vi "Generate Error.vi"(0 "Application in":refnum<class "Application.lvclass">, 5 "error in (no error)":errorcluster) -> (14 "Application out":refnum<class "Application.lvclass">)   [LabVIEW 2019, in "Application.lvclass"]
uses:
  Application.lvclass
  ErrorEvent.ctl
  Application.lvclass/Application.ctl
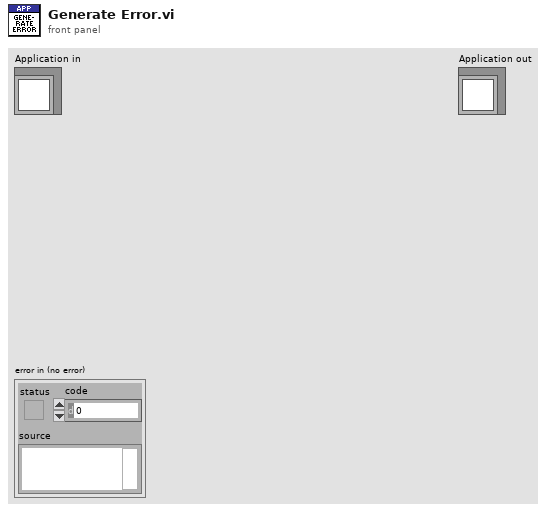
[diagram p1: front panel]
types:
  T1 = typedef "Application.lvclass/ErrorEvent.ctl" = cluster{"VI":string, "Time Stamp":timestamp, "Error":errorcluster, "Fatal":bool}
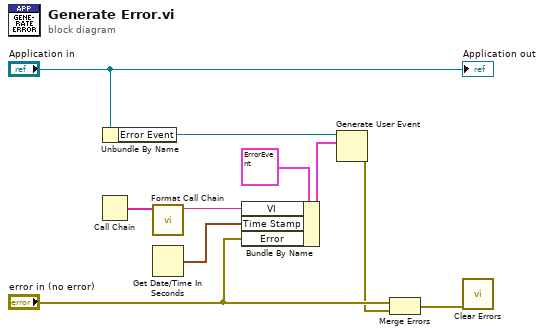
[diagram p0: block diagram]
diagram:
  n1 = Call Chain() -> (call chain=w3:string[])
  n2 = Unbundle By Name("Application in") -> ("Error Event"=w9:refnum<user-event>)
  n3 = call "Format Call Chain.vi"("Call Chain Array"=w3) -> ("Calling VI"=w2:string)  [unwired: 10 in]
  n4 = Get Date/Time In Seconds() -> (seconds since 1Jan1904=w4:timestamp)
  n5 = Bundle By Name(cluster=T1 {"VI"="", "Time Stamp"=timestamp(0 s since 1904-01-01), "Error"={"status"=FALSE, "code"=0, "source"=""}, "Fatal"=FALSE} ("event data"), "VI"=w2, "Time Stamp"=w4, "Error"="error in (no error)") -> (w5:T1)
  n6 = Generate User Event(user event=w9, event data cluster=w5) -> (error out=w6:errorcluster)  [unwired: 2 in, 1 out]
  n7 = Merge Errors("error in (no error)", w6) -> (w1:errorcluster)
  n8 = call <vilib>:"Clear Errors.vi"("error in (no error)"=w1) -> ()  [unwired: 5 in, 2 out]
  "Application out" <- "Application in"
